vi "_RT_ControlLoop_Param.vi"(8 "error in (no error)":errorcluster) -> ()   [LabVIEW 2016]
uses:
  PublicSubVI/Ctl/_ctl_MassAnal_ParamType.ctl
  PublicSubVI/Ctl/_ctl_RT_ParamDataCluster.ctl
  PublicSubVI/Ctl/_ctl_RT_FPGA_Function.ctl
  PublicSubVI/Ctl/_ctl_RT_CMD.ctl
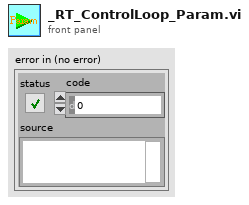
[diagram p1: front panel]
types:
  T1 = typedef "_ctl_MassAnal_ParamType.ctl" = enum16{"EventScript", "DO", "ExtAO"}
  T2 = typedef "_ctl_MassAnal_ParamType.ctl" = enum16{"Presets", "Ion guide & ion gate", "Events & param"}
  T3 = typedef "_ctl_RT_FPGA_Function.ctl" = enum16{"Initialisation", "Write AO", "Write DO", "Read AIs", "Read DIs", "Write ion guide & ion gate", "Presets", "Execution", "Read chasis temp"}
  T4 = typedef "_ctl_RT_FPGA_Function.ctl" = enum16{"Initialisation", "Execution", "Digital In"}
  T5 = typedef "_ctl_RT_ParamDataCluster.ctl" = cluster{"Type of Var":T1, "Data":variant}
  T6 = typedef "_ctl_RT_CMD.ctl" = cluster{"Cmd":string, "Data":variant, "Timestamp":timestamp}
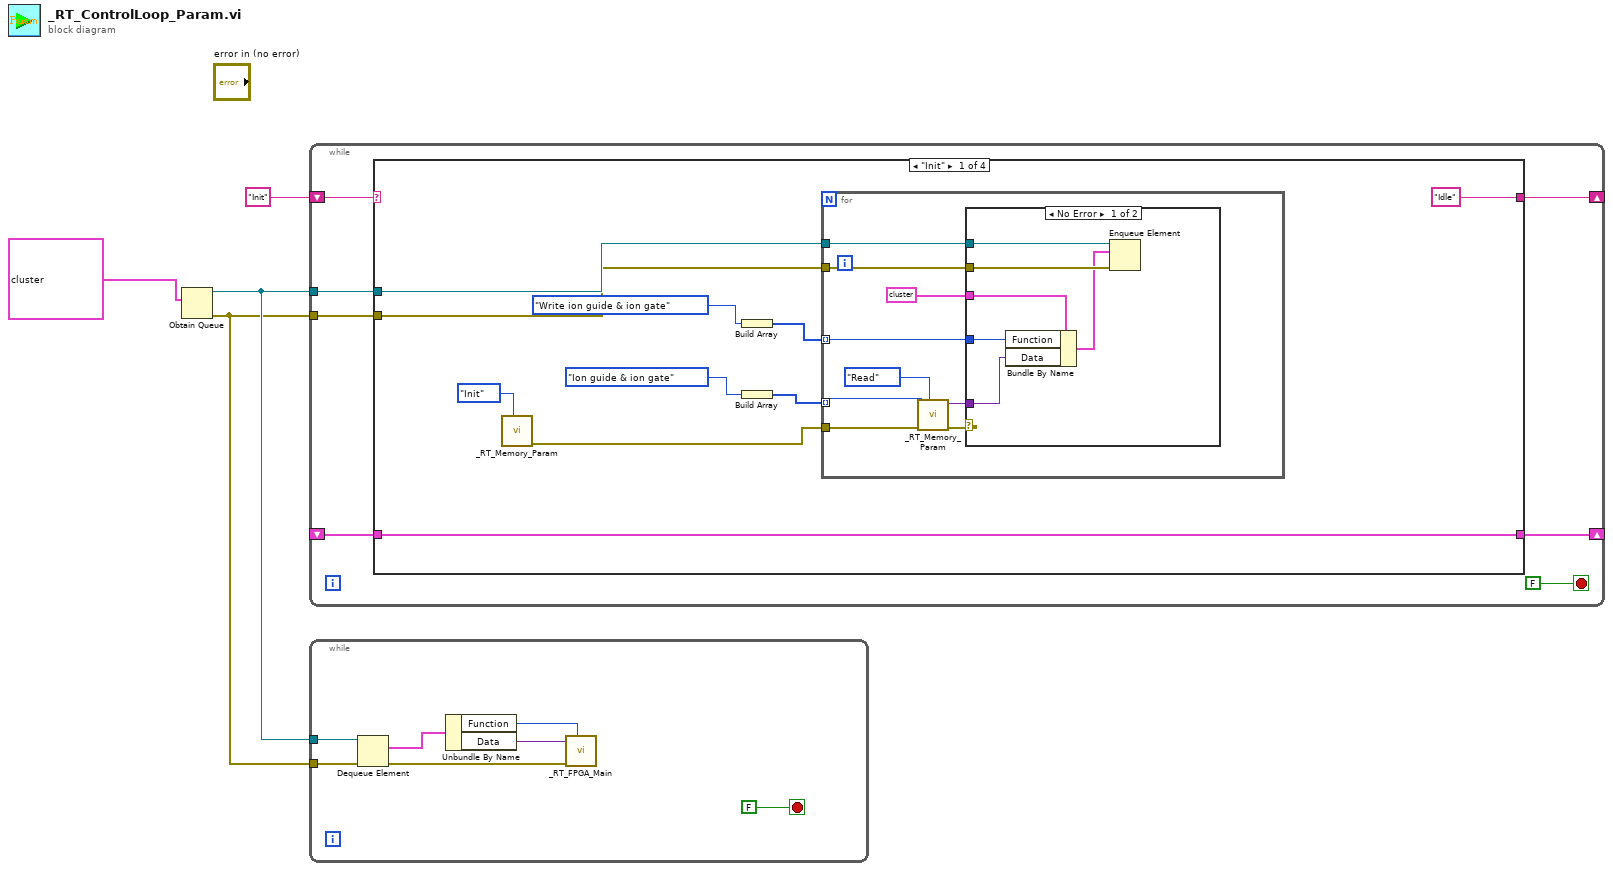
[diagram p0: block diagram]
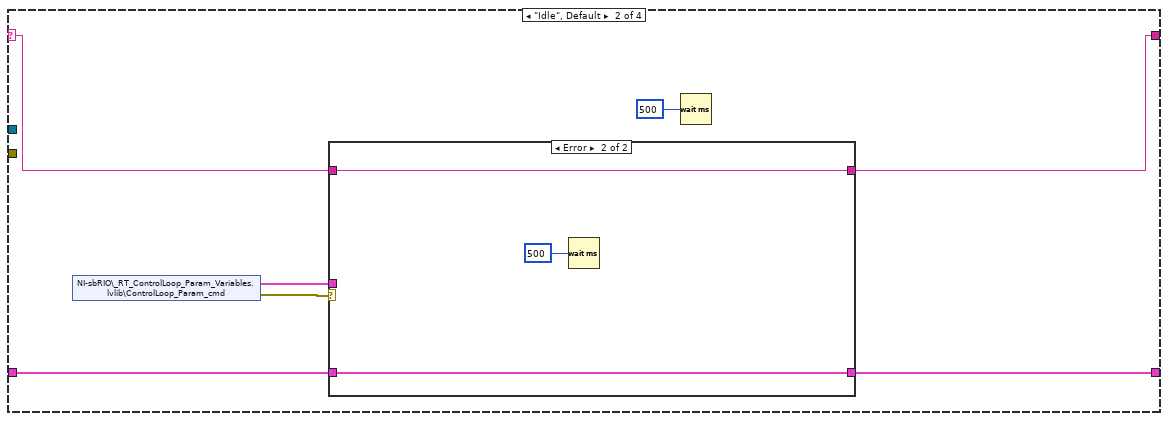
[diagram p3: hidden frame]
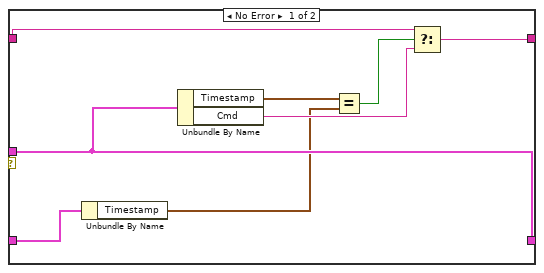
[diagram p4: hidden frame]
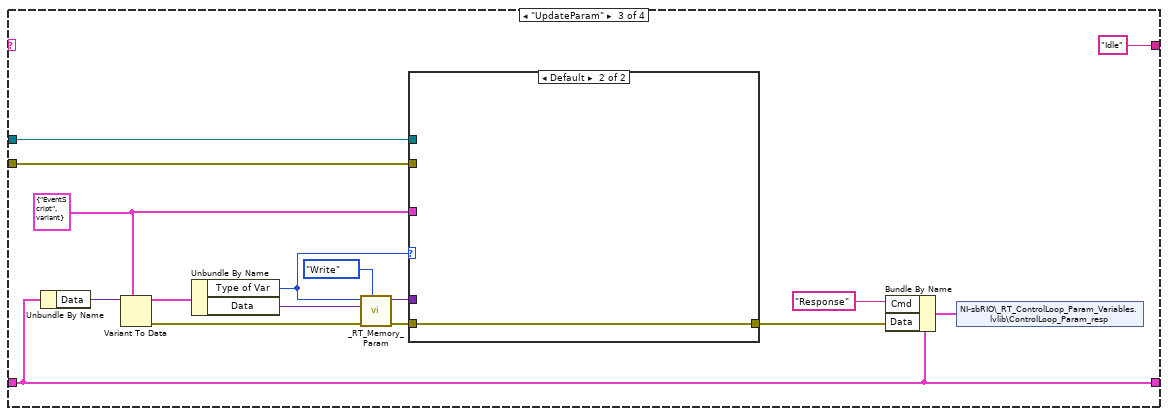
[diagram p5: hidden frame]
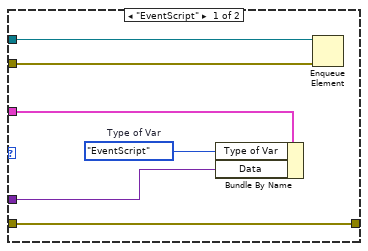
[diagram p6: hidden frame]
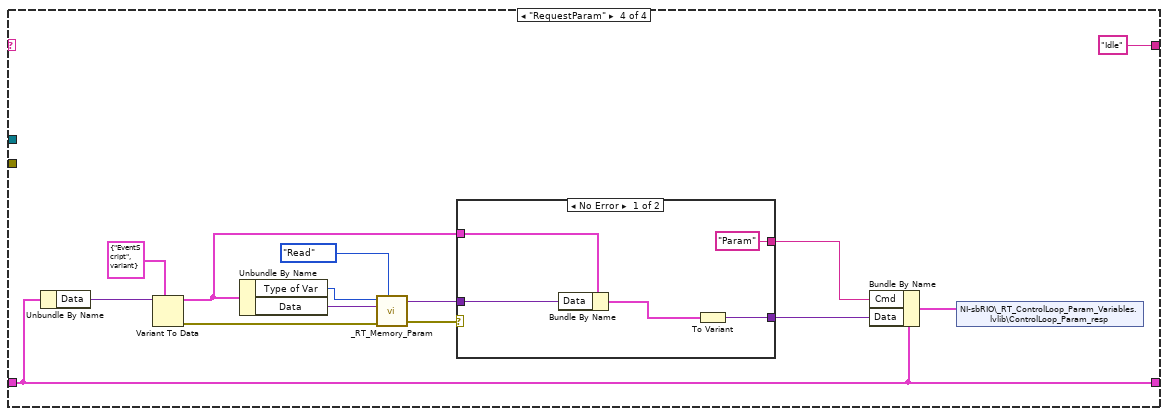
[diagram p7: hidden frame]
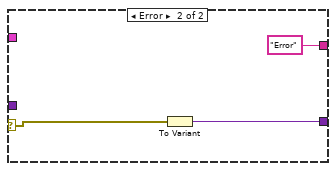
[diagram p8: hidden frame]
diagram:
  n1 = Obtain Queue(element data type=cluster{"Data":variant, "Type of Var":T1} {"Data"=variant, "Type of Var"=enum."EventScript"}) -> (queue out=w2:refnum<queue>, error out=w1:errorcluster)  [unwired: 4 in, 1 out]
  n2 = while {
    shift-right: [w10] -> _
    shift-left: "Init" -> [w11]
    shift-right: [w9] -> _
    shift-left: _ -> [w8]
    tunnel: w2 -> [w6]
    tunnel: w1 -> [w5]
    stop <- FALSE stop-if-true
    n3 = case shown="\"Init\"" w11 {
      selector: w11 -> [_ w43 _ _]
      tunnel: ["Idle" w42 "Idle" ("f") "Idle" ("f")] -> w10
      tunnel: [w19 w38 w56 w78] -> w9
      tunnel: w8 -> [w19 w37 w56 w78]
      tunnel: w6 -> [w13 _ w59 _]
      tunnel: w5 -> [w12 _ w58 _]
      frame "Init" {
        n4 = call "_RT_Memory_Param.vi"("Function"=enum16{"Write", "Init", "Read"}."Init") -> ("Error out"=w16:errorcluster)  [unwired: 9 in, 1 out]
        n5 = Build Array(_ctl_RT_FPGA_Function."Write ion guide & ion gate" ("Function")) -> (w17:T3[])
        n6 = Build Array(_ctl_MassAnal_ParamType."Ion guide & ion gate" ("Type of Var")) -> (w14:T2[])
        n7 = for {
          tunnel: w17 -> [w22] mode=indexing
          tunnel: w16 -> [w30]
          tunnel: w14 -> [w28] mode=indexing
          tunnel: w13 -> [w26]
          tunnel: w12 -> [w25]
          n8 = call "_RT_Memory_Param.vi"("Function"=enum16{"Write", "Init", "Read"}."Read", "Error in"=w30, "Type of Var"=w28) -> ("Error out"=w27:errorcluster, "Data out"=w23:variant)  [unwired: 7 in]
          n9 = case shown="No Error" w27 {
            tunnel: w26 -> [w36 _]
            tunnel: w25 -> [w35 _]
            tunnel: cluster{"Data":variant, "Function":T4} {"Data"=variant, "Function"=enum."Initialisation"} ("element") -> [w34 _]
            tunnel: w23 -> [w32 _]
            tunnel: w22 -> [w31 _]
            frame No Error {
              n10 = Bundle By Name(cluster=w34, "Function"=w31, "Data"=w32) -> (w33:cluster{"Data":variant, "Function":T4})
              n11 = Enqueue Element(queue=w36, element=w33, error in (no error)=w35) -> ()  [unwired: 1 in, 3 out]
            }
            frame Error {
            }
          }
        }
      }
      frame "Idle", Default {
        n12 = shared-variable "NI-sbRIO\\_RT_ControlLoop_Param_Variables.lvlib\\ControlLoop_Param_cmd"() -> (w41:T6, error out=w40:errorcluster)  [unwired: 1 in]
        n13 = case shown="Error" w40 {
          tunnel: w43 -> [w49 w54]
          tunnel: [w48 w54] -> w42
          tunnel: w41 -> [w46 _]
          tunnel: [w46 w52] -> w38
          tunnel: w37 -> [w45 w52]
          frame No Error {
            n14 = Unbundle By Name(w45) -> ("Timestamp"=w44:timestamp)
            n15 = Unbundle By Name(w46) -> ("Timestamp"=w51:timestamp, "Cmd"=w47:string)
            n16 = Equal?(x=w51, y=w44) -> (x = y?=w50:bool)
            n17 = Select(t=w49, s=w50, f=w47) -> (s? t:f=w48:string)
          }
          frame Error {
            n18 = Wait (ms)(milliseconds to wait=u32 500) -> ()  [unwired: 1 out]
          }
        }
        n19 = Wait (ms)(milliseconds to wait=u32 500 ("millisecond multiple")) -> ()  [unwired: 1 out]
      }
      frame "UpdateParam" {
        w55 = T5 {"Type of Var"=enum."EventScript", "Data"=variant}
        n20 = Unbundle By Name(w56) -> ("Data"=w69:variant)
        n21 = Variant To Data(type=w55, Variant=w69) -> (data=w67:T5, error out=w68:errorcluster)  [unwired: 1 in]
        n22 = Unbundle By Name(w67) -> ("Type of Var"=w65:T1, "Data"=w66:variant)
        n23 = call "_RT_Memory_Param.vi"("Function"=enum16{"Write", "Init", "Read"}."Write", "Error in"=w68, "Data in"=w66, "Type of Var"=w65) -> ("Error out"=w63:errorcluster, "Data out"=w64:variant)  [unwired: 6 in]
        n24 = case shown="Default" w65 {
          tunnel: w64 -> [w75 _]
          tunnel: w63 -> [w72 w77]
          tunnel: [w72 w77] -> w60
          tunnel: w59 -> [w74 _]
          tunnel: w55 -> [w76 _]
          tunnel: w58 -> [w73 _]
          frame "EventScript" {
            w71 = _ctl_MassAnal_ParamType."EventScript"  # Type of Var
            n25 = Bundle By Name(cluster=w76, "Type of Var"=w71, "Data"=w75) -> ()  [unwired: 1 out]
            n26 = Enqueue Element(queue=w74, error in (no error)=w73) -> ()  [unwired: 2 in, 3 out]
          }
          frame Default {
          }
        }
        n27 = Bundle By Name(cluster=w56, "Cmd"="Response", "Data"=w60) -> (w61:T6)
        n28 = shared-variable "NI-sbRIO\\_RT_ControlLoop_Param_Variables.lvlib\\ControlLoop_Param_resp"(w61) -> ()  [unwired: 1 in, 1 out]
      }
      frame "RequestParam" {
        n29 = Unbundle By Name(w78) -> ("Data"=w90:variant)
        n30 = Variant To Data(type=T5 {"Type of Var"=enum."EventScript", "Data"=variant}, Variant=w90) -> (data=w79:T5, error out=w89:errorcluster)  [unwired: 1 in]
        n31 = Unbundle By Name(w79) -> ("Type of Var"=w87:T1, "Data"=w88:variant)
        n32 = call "_RT_Memory_Param.vi"("Function"=enum16{"Write", "Init", "Read"}."Read", "Error in"=w89, "Data in"=w88, "Type of Var"=w87) -> ("Error out"=w80:errorcluster, "Data out"=w84:variant)  [unwired: 6 in]
        n33 = case shown="No Error" w80 {
          selector: w80 -> [_ w99]
          tunnel: w84 -> [w96 _]
          tunnel: [w93 w97] -> w83
          tunnel: ["Param" ("Cmd") "Error" ("Cmd")] -> w81
          tunnel: w79 -> [w92 _]
          frame No Error {
            n34 = Bundle By Name(cluster=w92, "Data"=w96) -> (w95:T5)
            n35 = To Variant(anything=w95) -> (Variant=w93:variant)
          }
          frame Error {
            n36 = To Variant(anything=w99) -> (Variant=w97:variant)
          }
        }
        n37 = Bundle By Name(cluster=w78, "Cmd"=w81, "Data"=w83) -> (w85:T6)
        n38 = shared-variable "NI-sbRIO\\_RT_ControlLoop_Param_Variables.lvlib\\ControlLoop_Param_resp"(w85) -> ()  [unwired: 1 in, 1 out]
      }
    }
  }
  n39 = while {
    tunnel: w2 -> [w106]
    tunnel: w1 -> [w105]
    stop <- FALSE stop-if-true
    n40 = Dequeue Element(queue=w106, error in (no error)=w105) -> (element=w104:cluster{"Data":variant, "Type of Var":T1}, error out=w101:errorcluster)  [unwired: 1 in, 2 out]
    n41 = Unbundle By Name(w104) -> ("Function"=w102:T4, "Data"=w103:variant)
    n42 = call "_RT_FPGA_Main.vi"("Function"=w102, "Error in"=w101, "Data_in"=w103) -> ()  [unwired: 6 in, 3 out]
  }
